vi "ASK_DeModulation.vi"() -> ()   [LabVIEW 2015]
panel:
  out "Demodulated Square":dbl(graph)
  out "Output Chart":dbl(graph)
  out "Modulating Square Chart":i8(graph)
  in  "stop":bool
  in  "Number of Cycles":i32
  in  "number of levels":dbl
  in  "Carrier Frequency":i32
  in  "Sampling freq.":i32
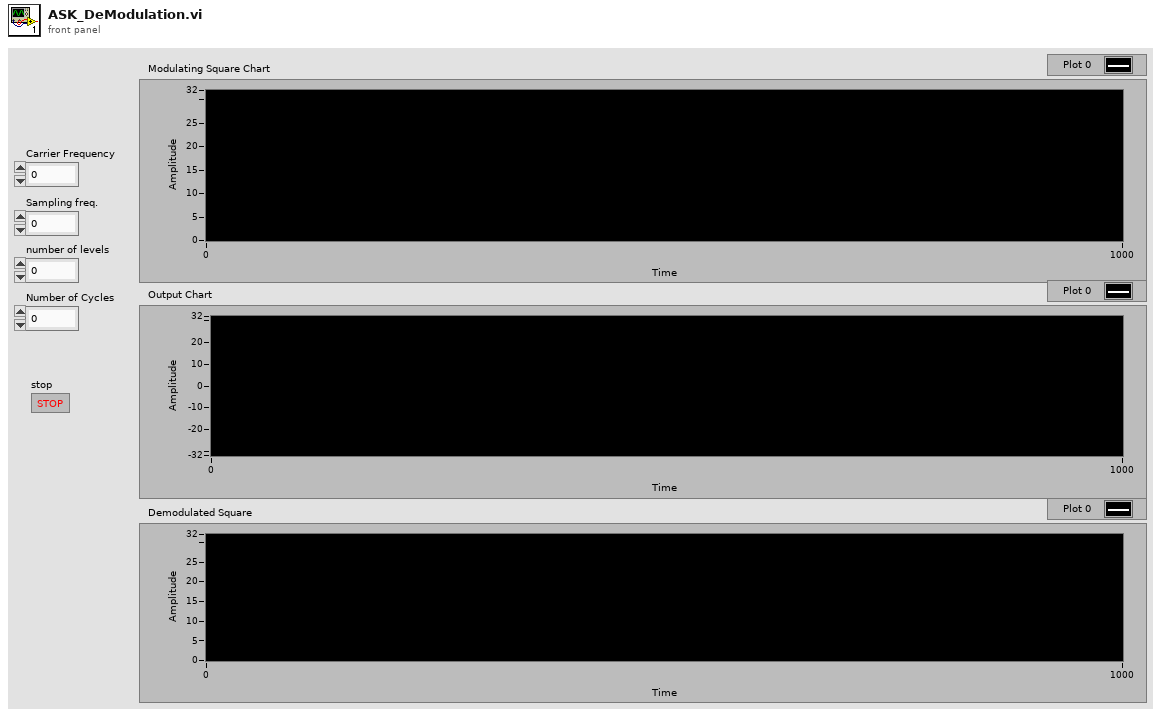
[diagram p1: front panel]
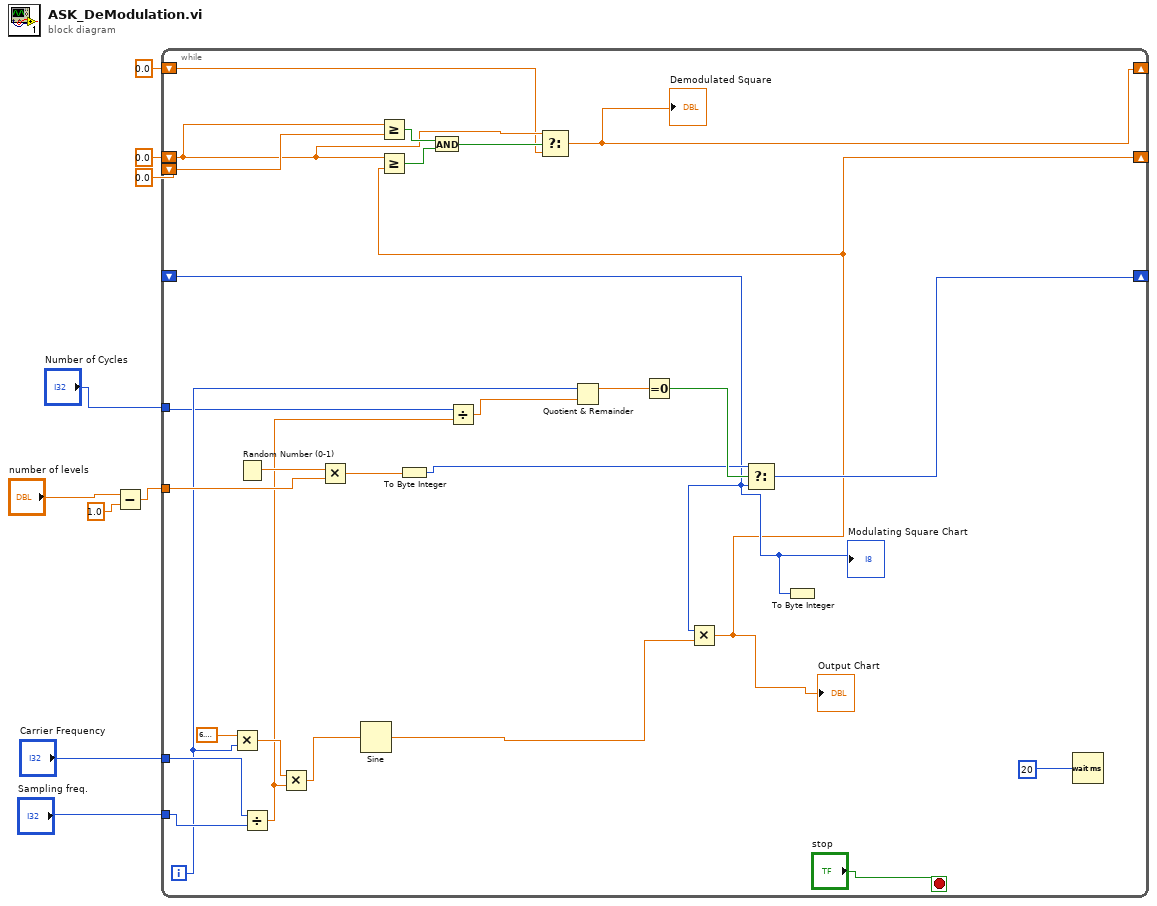
[diagram p0: block diagram]
diagram:
  n1 = Subtract(x="number of levels", y=1.0) -> (x-y=w4:dbl)
  n2 = while {
    tunnel: "Sampling freq." -> [w37]
    tunnel: "Carrier Frequency" -> [w26]
    tunnel: w4 -> [w34]
    shift-right: [w28] -> _
    shift-left: _ -> [w19]
    tunnel: "Number of Cycles" -> [w24]
    shift-right: [w16] -> _
    shift-left: 0.0 -> [w12]
    shift-left: 0.0 -> [w17]
    shift-right: [w10] -> _
    shift-left: 0.0 -> [w11]
    i -> [w25]
    stop <- "stop" stop-if-true
    n3 = Multiply(x=6.283185307179586, y=w25) -> (x*y=w32:dbl)
    n4 = Random Number (0-1)() -> (number: 0 to 1=w35:dbl)
    n5 = Divide(x=w26, y=w37) -> (x/y=w23:dbl)
    n6 = Multiply(x=w32, y=w23) -> (x*y=w36:dbl)
    n7 = Multiply(x=w35, y=w34) -> (x*y=w33:dbl)
    n8 = Sine(x=w36) -> (sin(x)=w18:dbl)
    n9 = Greater Or Equal?(x=w12, y=w17) -> (x >= y?=w15:bool)
    n10 = To Byte Integer(number=w33) -> (8bit integer=w29:i8)
    n11 = Divide(x=w24, y=w23) -> (x/y=w22:dbl)
    n12 = Quotient & Remainder(x=w25, y=w22) -> (x-y*floor(x/y)=w31:dbl)  [unwired: 1 out]
    n13 = Equal To 0?(x=w31) -> (x = 0?=w30:bool)
    n14 = Multiply(x=w19, y=w18) -> (x*y=w16:dbl)
    "Output Chart" <- w16
    n15 = Greater Or Equal?(x=w12, y=w16) -> (x >= y?=w14:bool)
    n16 = And(x=w15, y=w14) -> (x .and. y?=w13:bool)
    n17 = Select(t=w12, s=w13, f=w11) -> (s? t:f=w10:dbl)
    "Demodulated Square" <- w10
    n18 = Select(t=w29, s=w30, f=w19) -> (s? t:f=w28:i8)
    n19 = To Byte Integer(number=w19) -> ()  [unwired: 1 out]
    n20 = Wait (ms)(milliseconds to wait=u32 20) -> ()  [unwired: 1 out]
    "Modulating Square Chart" <- w19
  }
